vi "Generate File.vi"(11 "file path (use dialog)":path=path "C:/Users/Administrator/Desktop/Temp/Shared Memory Groups/C Header Generator/test.h") -> ()   [LabVIEW 2013, in "C Header Generator.lvlib"]
uses:
  C Header Generator.lvlib
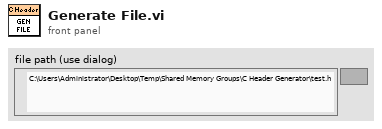
[diagram p1: front panel]
types:
  T1 = enum16{"open", "replace", "create", "open or create", "replace or create", "replace or create with confirmation"}
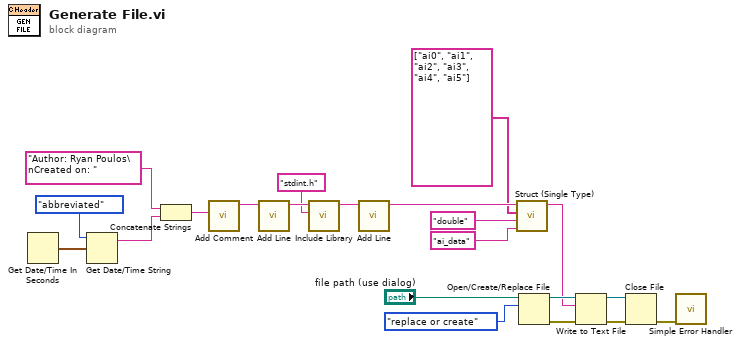
[diagram p0: block diagram]
diagram:
  n1 = Get Date/Time In Seconds() -> (seconds since 1Jan1904=w11:timestamp)
  n2 = Get Date/Time String(date format (0)=enum16{"short", "long", "abbreviated"}."abbreviated", seconds (now)=w11) -> (date string=w1:string)  [unwired: 1 in, 1 out]
  n3 = Concatenate Strings("Author: Ryan Poulos\nCreated on: ", w1) -> (w2:string)
  n4 = call "Add Comment.vi"("Comment"=w2) -> ("String out"=w3:string)  [unwired: 10 in]
  n5 = call "Add Line.vi"("String in"=w3) -> ("String out"=w9:string)  [unwired: 10 in]
  n6 = call "Include Library.vi"("Library Name"="stdint.h", "String in"=w9) -> ("String out"=w13:string)  [unwired: 9 in]
  n7 = call "Add Line.vi"("String in"=w13) -> ("String out"=w12:string)  [unwired: 10 in]
  n8 = call "Struct (Single Type).vi"("Struct name"="ai_data" ("Typedef name"), "Data type"="double", "Variable names"=string[] ["ai0", "ai1", "ai2", "ai3", "ai4", "ai5"], "String in"=w12) -> ("String out"=w17:string)  [unwired: 7 in]
  n9 = Open/Create/Replace File(file path (use dialog)="file path (use dialog)", operation (0:open)=T1."replace or create") -> (refnum out=w19:refnum<file>, error out=w18:errorcluster)  [unwired: 4 in, 1 out]
  n10 = Write to Text File(file (use dialog)=w19, text=w17, error in=w18) -> (refnum out=w15:refnum<file>, error out=w16:errorcluster)  [unwired: 1 in, 1 out]
  n11 = Close File(refnum=w15, error in=w16) -> (error out=w14:errorcluster)  [unwired: 1 out]
  n12 = call <vilib>:"Simple Error Handler.vi"("error in (no error)"=w14) -> ()  [unwired: 4 in, 5 out]
